vi "Reset Menu Button.vi"(8 "error in (no error)":errorcluster, 11 "MenuButton in":refnum<class "MenuButton.lvclass">) -> (0 "error out":errorcluster, 3 "MenuButton out":refnum<class "MenuButton.lvclass">)   [LabVIEW 2017, in "MenuButtons.lvlib" / "MenuButton.lvclass"]
uses:
  MenuButton.lvclass
  MenuButton.lvclass/MenuButton.ctl
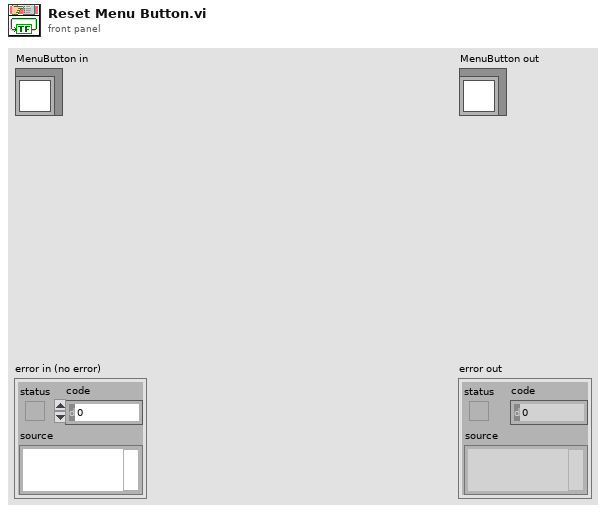
[diagram p1: front panel]
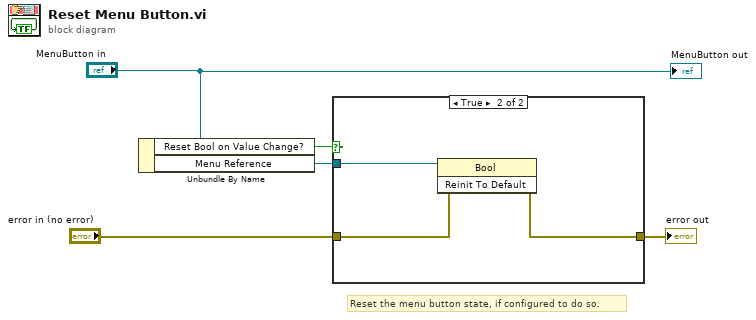
[diagram p0: block diagram]
diagram:
  # "Reset the menu button state, if configured to do so."
  n1 = Unbundle By Name("MenuButton in") -> ("Reset Bool on Value Change?"=w4:bool, "Menu Reference"=w3:refnum<vi>)
  n2 = case shown="True" w4 {
    tunnel: w3 -> [_ w9]
    tunnel: "error in (no error)" -> [w6 w8]
    tunnel: [w6 w7] -> w1
    frame False {
    }
    frame True {
      n3 = invoke class="Bool" method="Reinit To Default"(reference=w9, error in=w8) -> (error out=w7:errorcluster)  [unwired: 1 in, 2 out]
    }
  }
  "error out" <- w1
  "MenuButton out" <- "MenuButton in"
